vi "Calcolo Hrif.vi"(6 "Nmisure Hrif":i8, 7 "CALCOLA SU N MIS":bool, 8 "HTOT REF":dbl, 9 "Pto NPSH":u8, 10 "indici":T1, 11 "Tabella":string[][](array[string])) -> (2 "Hrif":dbl, 3 "Tabella":string[][](array[string]))   [LabVIEW 2019]
uses:
  TypeDef/Indici.ctl
  <vilib>/Analysis/baseanly.llb/Mean (DBL).vi
  <vilib>/Analysis/NI_AALBase.lvlib
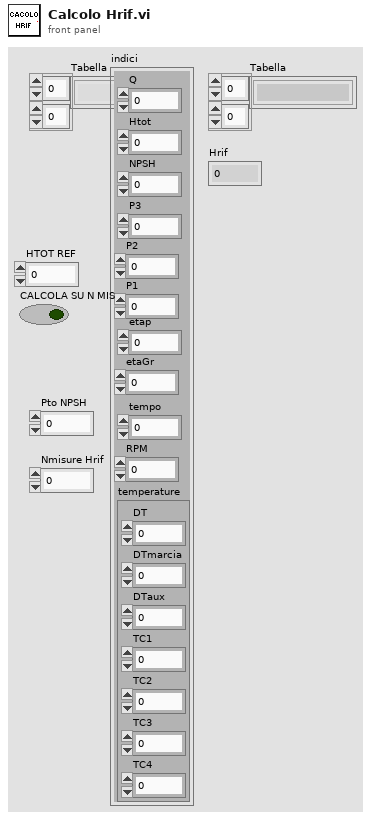
[diagram p1: front panel]
types:
  T1 = typedef "Indici.ctl" = cluster{"Q":i32, "Htot":i32, "NPSH":i32, "P3":i32, "etap":i32, "temperature":cluster{"DT":i32, "DTmarcia":i32, "DTaux":i32, "TC1":i32, "TC2":i32, "TC3":i32, "TC4":i32}, "tempo":i32, "P2":i32, "P1":i32, "etaGr":i32, "RPM":i32}
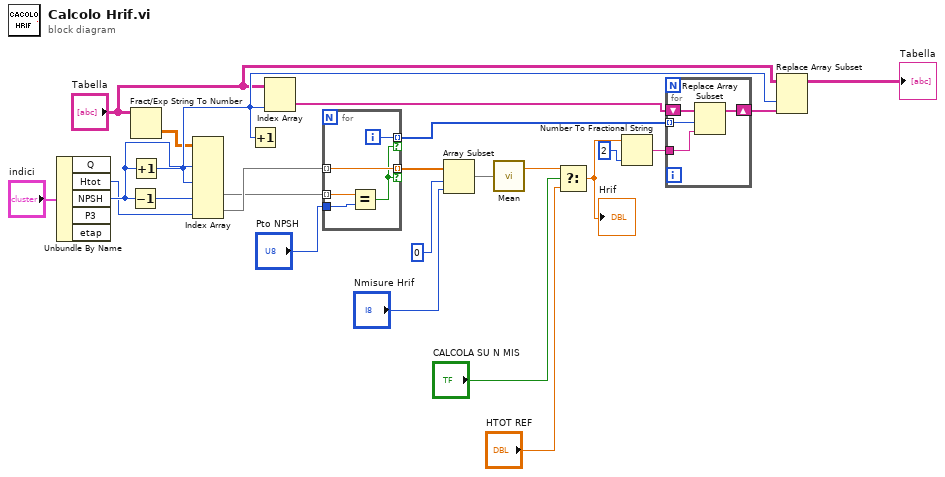
[diagram p0: block diagram]
diagram:
  n1 = Unbundle By Name("indici") -> ("Htot"=w6:i32, "NPSH"=w8:i32)  [unwired: 3 out]
  n2 = Decrement(x=w8) -> (x-1=w7:i32)
  n3 = Fract/Exp String To Number(string="Tabella") -> (number=w9:dbl[][])  [unwired: 3 in, 1 out]
  n4 = Increment(x=w8) -> (x+1=w21:i32)
  n5 = Index Array(array=w9, index (col) #1=w8, index (col) #2=w21, index (col) #3=w7, index (col) #4=w6) -> (element #3=w11:dbl[], element #4=w14:dbl[])  [unwired: 4 in, 2 out]
  n6 = Increment(x=w21) -> ()  [unwired: 1 out]
  n7 = Index Array(array="Tabella", index (col)=w21) -> (element=w17:string[])  [unwired: 1 in]
  n8 = for {
    tunnel: "Pto NPSH" -> [w28]
    tunnel: w11 -> [w29] mode=indexing
    tunnel: [w27] -> w15 mode=indexing if=w25
    tunnel: w14 -> [w27] mode=indexing
    tunnel: [w26] -> w18 mode=indexing if=w25
    i -> [w26]
    n9 = Equal?(x=w29, y=w28) -> (x = y?=w25:bool)
  }
  n10 = Array Subset(array=w15, index=0, length="Nmisure Hrif") -> (w13:dbl[])
  n11 = call-poly <vilib>:"Mean.vi"("X"=w13) -> ("mean"=w4:dbl)  [unwired: 1 out]
  n12 = Select(t=w4, s="CALCOLA SU N MIS", f="HTOT REF") -> (s? t:f=w1:dbl)
  "Hrif" <- w1
  n13 = Number To Fractional String(number=w1, precision (6)=i16 2) -> (F-format string=w19:string)  [unwired: 2 in]
  n14 = for {
    shift-right: [w32] -> w22
    shift-left: w17 -> [w33]
    tunnel: w18 -> [w31] mode=indexing
    tunnel: w19 -> [w30]
    n15 = Replace Array Subset(array=w33, new element=w30, index=w31) -> (w32:string[])
  }
  n16 = Replace Array Subset "Replace Array Subset"(array="Tabella", new element=w22, index (col)=w21) -> (→"Tabella":string[][])  [unwired: 1 in]
